vi "Save Stats (Attach).vi"(0 "Filepath":path, 3 "Data":string[][](array[string]), 11 "Error In":errorcluster) -> (4 "xlRefs":T1, 15 "Error Out":errorcluster)   [LabVIEW 2013]
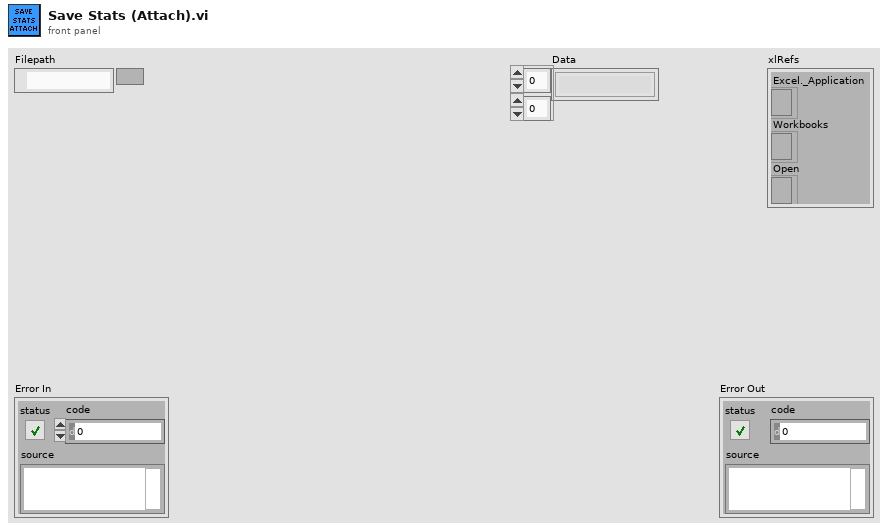
[diagram p1: front panel]
types:
  T1 = cluster{"Excel._Application":refnum<k7>, "Workbooks":refnum<k7>, "Open":refnum<k7>}
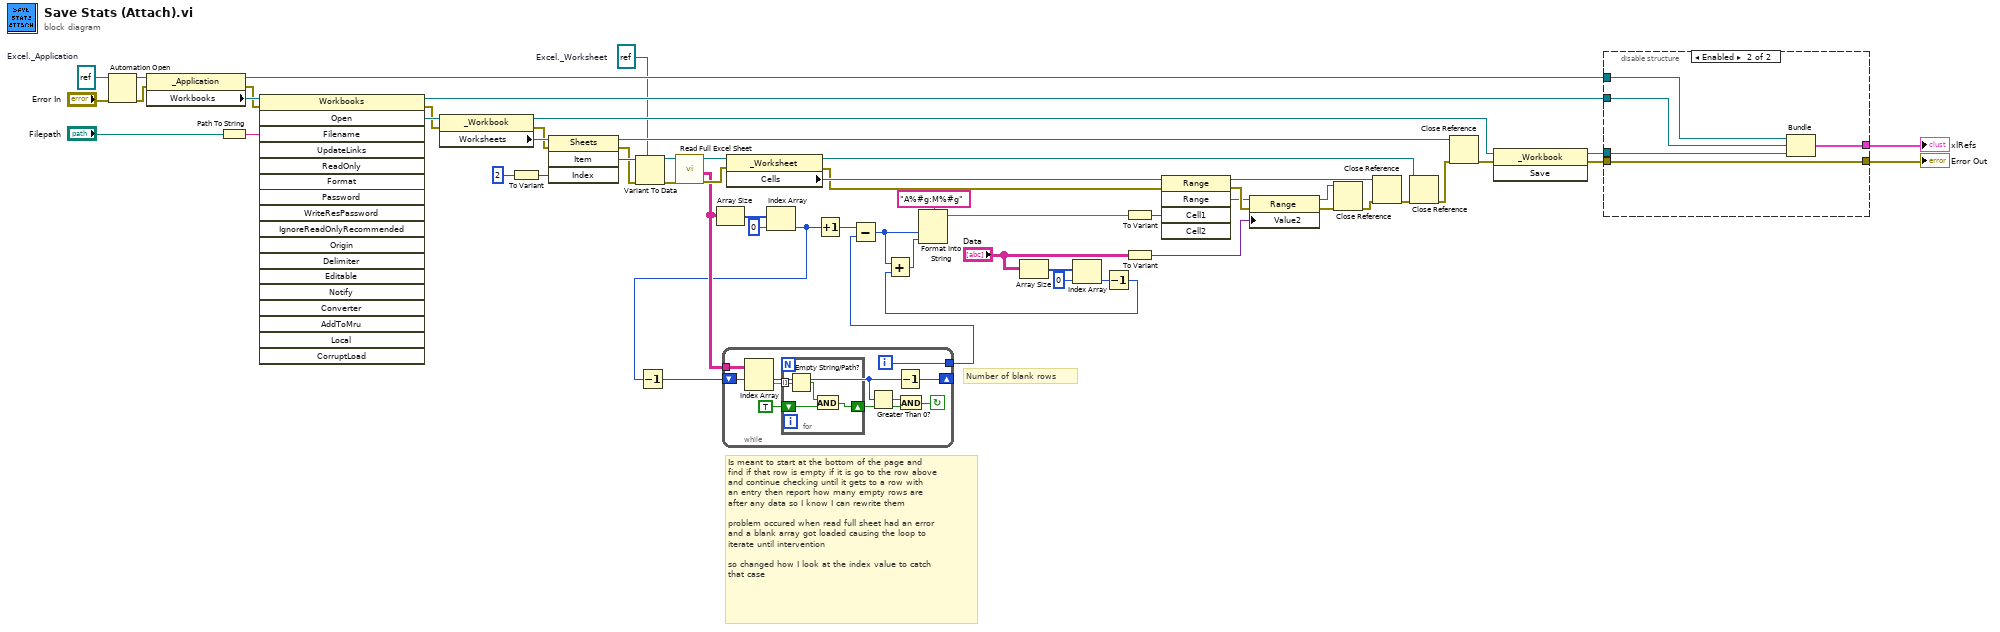
[diagram p0: block diagram]
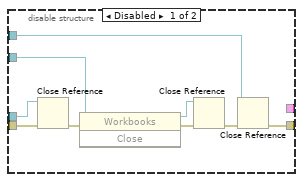
[diagram p2: hidden frame]
diagram:
  w43 = refnum<k7> refnum  # Excel._Worksheet
  w56 = refnum<k7> refnum  # Excel._Application
  # "Is meant to start at the bottom of the page and\nfind if that row is empty if it is go to the row above\nand continue checking until it gets to a row with\nan entry then report how many empty rows are\nafter any data so I know I can rewrite them\n\nproblem occured when read full sheet had an error\nand a blank array got loaded causing the loop to \niterate until intervention\n\nso changed how I look at the index value to catch\nthat case"
  # "Number of blank rows"
  n1 = Automation Open(error in (no error)="Error In", Automation Refnum=w56) -> (Automation Refnum=w57:refnum<k7>, error out=w58:errorcluster)  [unwired: 2 in]
  n2 = property class="_Application"(reference=w57, error in=w58) -> (reference out=w52:refnum<k7>, error out=w53:errorcluster, "Workbooks"=w59:refnum<k7>)
  n3 = Path To String(path="Filepath") -> (string=w49:string)
  n4 = invoke class="Workbooks" method="Open"(reference=w59, error in=w53, "Filename"=w49) -> (reference out=w54:refnum<k7>, error out=w51:errorcluster, "Open"=w55:refnum<k7>)  [unwired: 15 in, 15 out]
  n5 = property class="_Workbook"(reference=w55, error in=w51) -> (reference out=w46:refnum<k7>, error out=w22:errorcluster, "Worksheets"=w23:refnum<k7>)
  n6 = To Variant(anything=2) -> (Variant=w38:variant)
  n7 = invoke class="Sheets" method="Item"(reference=w23, error in=w22, "Index"=w38) -> (reference out=w44:refnum<k7>, error out=w36:errorcluster, "Item"=w37:variant)  [unwired: 1 in, 1 out]
  n8 = Variant To Data(error in=w36, type=w43, Variant=w37) -> (data=w16:refnum<k7>, error out=w15:errorcluster)
  n9 = call "Read Full Excel Sheet.vi"("Error In"=w15, "Excel._Worksheet"=w16) -> ("Error Out"=w14:errorcluster, "Data"=w12:string[][], "Reference Out"=w17:refnum<k7>)  [unwired: 7 in]
  n10 = Array Size(array=w12) -> (size(s)=w21:i32[])
  n11 = property class="_Worksheet"(reference=w17, error in=w14) -> (reference out=w34:refnum<k7>, error out=w18:errorcluster, "Cells"=w19:refnum<k7>)
  n12 = Index Array(array=w21, index=0) -> (element=w8:i32)
  n13 = Decrement(x=w8) -> (x-1=w11:i32)
  n14 = while {
    tunnel: w12 -> [w68]
    tunnel: [w65] -> w10
    shift-right: [w64] -> _
    shift-left: w11 -> [w63]
    i -> [w65]
    stop <- w60 continue-if-true
    n15 = Index Array(array=w68, index (row)=w63) -> (element=w66:string[])  [unwired: 1 in]
    n16 = for {
      tunnel: w66 -> [w72] mode=indexing
      shift-right: [w70] -> w61
      shift-left: TRUE -> [w69]
      n17 = Empty String/Path?(string/path=w72) -> (empty?=w71:bool)
      n18 = And(x=w71, y=w69) -> (x .and. y?=w70:bool)
    }
    n19 = Greater Than 0?(x=w63) -> (x > 0?=w62:bool)
    n20 = Decrement(x=w63) -> (x-1=w64:i32)
    n21 = And(x=w62, y=w61) -> (x .and. y?=w60:bool)
  }
  n22 = Increment(x=w8) -> (x+1=w7:i32)
  n23 = Subtract(x=w7, y=w10) -> (x-y=w9:i32)
  n24 = Array Size(array="Data") -> (size(s)=w6:i32[])
  n25 = Index Array(array=w6, index=0) -> (element=w4:i32)
  n26 = Decrement(x=w4) -> (x-1=w3:i32)
  n27 = Add(x=w9, y=w3) -> (x+y=w13:i32)
  n28 = Format Into String(format string="A%#g:M%#g", w9, w13) -> (resulting string=w25:string)  [unwired: 2 in, 1 out]
  n29 = To Variant(anything=w25) -> (Variant=w30:variant)
  n30 = To Variant(anything="Data") -> (Variant=w28:variant)
  n31 = invoke class="Range" method="Range"(reference=w19, error in=w18, "Cell1"=w30) -> (reference out=w33:refnum<k7>, error out=w29:errorcluster, "Range"=w24:refnum<k7>)  [unwired: 2 in, 2 out]
  n32 = property class="Range"(reference=w24, error in=w29, "Value2"=w28) -> (reference out=w27:refnum<k7>, error out=w26:errorcluster)
  n33 = Close Reference(reference=w27, error in (no error)=w26) -> (error out=w32:errorcluster)
  n34 = Close Reference(reference=w33, error in (no error)=w32) -> (error out=w35:errorcluster)
  n35 = Close Reference(reference=w34, error in (no error)=w35) -> (error out=w45:errorcluster)
  n36 = Close Reference(reference=w44, error in (no error)=w45) -> (error out=w50:errorcluster)
  n37 = invoke class="_Workbook" method="Save"(reference=w46, error in=w50) -> (reference out=w47:refnum<k7>, error out=w48:errorcluster)  [unwired: 1 in, 1 out]
  n38 = disable-structure shown="Enabled" {
    disable-tunnel: w54 -> [w80 w84]
    disable-tunnel: w52 -> [w77 w85]
    disable-tunnel: w48 -> [w75 w86]
    disable-tunnel: w47 -> [w74 w83]
    disable-tunnel: [w73 w86] -> w42
    disable-tunnel: [_ w82] -> w1
    frame Disabled {
      n39 = Close Reference(reference=w74, error in (no error)=w75) -> (error out=w76:errorcluster)
      n40 = invoke class="Workbooks" method="Close"(reference=w80, error in=w76) -> (reference out=w79:refnum<k7>, error out=w78:errorcluster)  [unwired: 1 in, 1 out]
      n41 = Close Reference(reference=w79, error in (no error)=w78) -> (error out=w81:errorcluster)
      n42 = Close Reference(reference=w77, error in (no error)=w81) -> (error out=w73:errorcluster)
    }
    frame Enabled {
      n43 = Bundle("Excel._Application"=w85, "Workbooks"=w84, "Open"=w83) -> (w82:T1)  [unwired: 1 in]
    }
  }
  "Error Out" <- w42
  "xlRefs" <- w1
